vi "Get Column Name.vi"(8 "error in (no error)":errorcluster, 11 "SQL Statement in":refnum<class "SQL Statement.lvclass">) -> (0 "error out":errorcluster, 2 "Column Name":string, 3 "SQL Statement out":refnum<class "SQL Statement.lvclass">)   [LabVIEW 2023, in "SQLiteSupport.lvlib" / "SQL Statement.lvclass"]
doc: "Returns the name assigned to the column in the result set of a SELECT statement."
uses:
  SQL Statement.lvclass
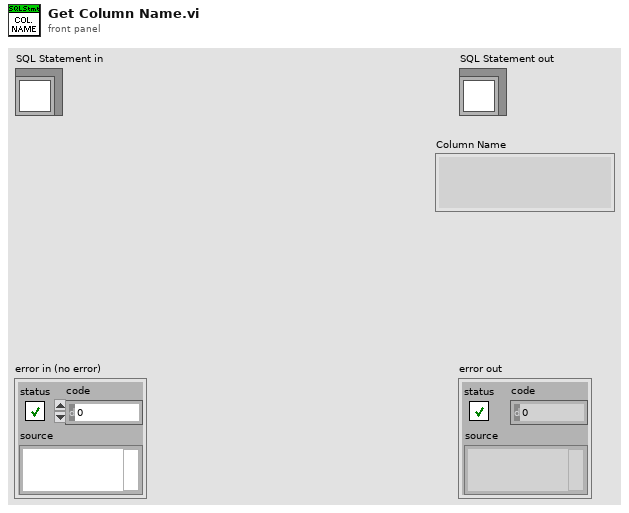
[diagram p1: front panel]
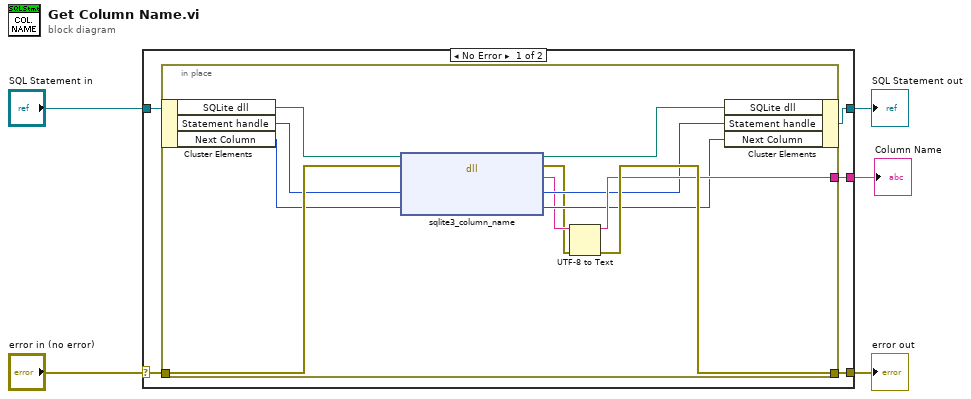
[diagram p0: block diagram]
diagram:
  n1 = case shown="No Error" "error in (no error)" {
    selector: "error in (no error)" -> [w10 w23]
    tunnel: [w9 w23] -> w4
    tunnel: [w6 w22] -> w2
    tunnel: "SQL Statement in" -> [w7 w22]
    tunnel: [w8 _] -> w1
    frame No Error {
      n2 = in-place {
        in-place-border: w10 -> [w21]
        in-place-border: [w20] -> w9
        in-place-border: [w19] -> w8
        n3 = in-place-cluster #1(w7) -> ("SQLite dll"=w16:path, "Statement handle"=w17:u64, "Next Column"=w18:i32)
        n4 = dll-call lib="C:/LabVIEW_JDP/Support/SQLite/SQL Connection/sqlite3.dll" fn="sqlite3_column_name"(path in=w16, error in=w21, "Statement"=w17, "Column"=w18) -> (path out=w13:path, error out=w11:errorcluster, "Text"=w12:string, "Statement"=w14:u64, "Column"=w15:i32)  [unwired: 1 in]
        n5 = UTF-8 to Text(8:w11, 11:w12) -> (0:w20:errorcluster, 3:w19:string)  [unwired: 1 in]
        n6 = in-place-cluster #1("SQLite dll"=w13, "Statement handle"=w14, "Next Column"=w15) -> (w6:refnum<class "SQL Statement.lvclass">)
      }
    }
    frame Error {
    }
  }
  "error out" <- w4
  "SQL Statement out" <- w2
  "Column Name" <- w1
